vi "Connected Hosts List.vi"(7 "Action":T1, 8 "error in":errorcluster, 11 "IP:Port:Master/Slave":string) -> (0 "error out":errorcluster, 2 "List of IP:Port:Master/Slave":string[](array[string]), 3 "IP:Port:Master/Slave out":string)   [LabVIEW 2021, in "RT Interpreter.lvlib"]
uses:
  RT Interpreter.lvlib
  Connected Hosts List Action--enum.ctl
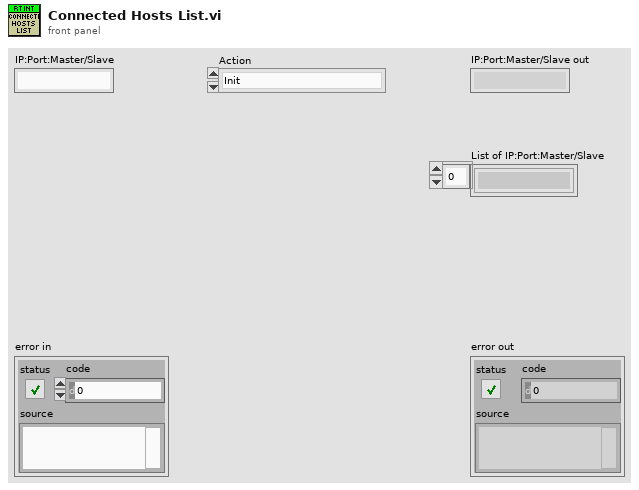
[diagram p1: front panel]
types:
  T1 = typedef "RT Interpreter.lvlib/Connected Hosts List Action--enum.ctl" = enum16{"Init", "Add Instance", "Remove Instance", "List Instances"}
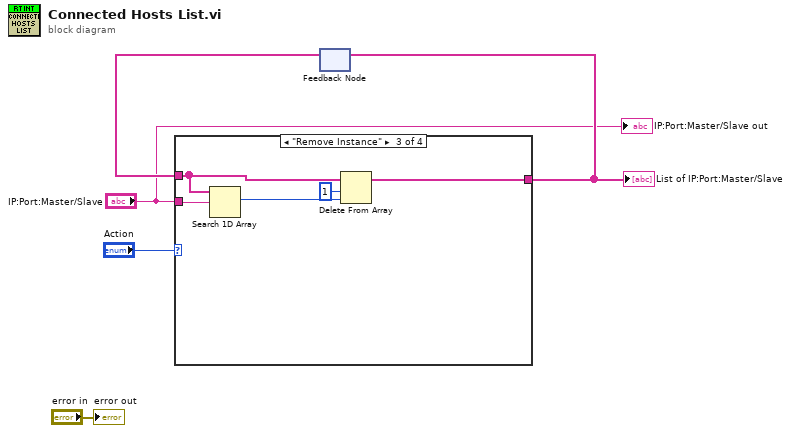
[diagram p0: block diagram]
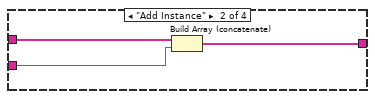
[diagram p3: hidden frame]
diagram:
  n1 = feedback #1() -> (w4:string[])  [unwired: 1 in]
  n2 = case shown="\"Remove Instance\"" "Action" {
    tunnel: "IP:Port:Master/Slave" -> [_ w6 w11 _]
    tunnel: [_ w7 w10 w14] -> w5
    tunnel: w4 -> [_ w8 w13 w14]
    frame "Init", Default {
    }
    frame "Add Instance" {
      n3 = Build Array (concatenate)(w8, w6) -> (w7:string[])
    }
    frame "Remove Instance" {
      n4 = Search 1D Array(1D array=w13, element=w11) -> (index of element=w9:i32)  [unwired: 1 in]
      n5 = Delete From Array(array=w13, length=1, index=w9) -> (array with subset deleted=w10:string[])  [unwired: 1 out]
    }
    frame "List Instances" {
    }
  }
  "List of IP:Port:Master/Slave" <- w5
  n6 = feedback-in #1(w5) -> ()
  "error out" <- "error in"
  "IP:Port:Master/Slave out" <- "IP:Port:Master/Slave"
